vi "config CANcoder.vi"(8 "error in (no error)":errorcluster, 11 "CANcoder init data":T1={"description"="", "Installed?"=FALSE, "CAN ID"=0, "CAN Bus"="", "refnum name"="", "Sensor Direction"=FALSE, "Magnet Offset (Degrees)"=0.0, "gear ratio"=1.0} {"gear ratio" format="%_5f"}) -> (0 "error out":errorcluster)   [LabVIEW 2023]
uses:
  ctrl defs/ctrl CANcoder.ctl
  <vilib>/Rock Robotics/WPI/ThirdParty/Phoenix-LabVIEW/CANCoder/Controls/CTRE_Phoenix_CANcoder_Configurables.ctl
  <vilib>/Rock Robotics/WPI/ThirdParty/Phoenix-LabVIEW/CANCoder/Controls/CTRE_Phoenix_CANcoder_SensorInitializationStrategy.ctl
  <vilib>/Rock Robotics/WPI/ThirdParty/Phoenix-LabVIEW/CANCoder/Controls/CTRE_Phoenix_CANcoder_AbsoluteSensorRange.ctl
  <vilib>/Rock Robotics/WPI/ThirdParty/Phoenix-LabVIEW/Motor Controller/Controls/CTRE_Phoenix_MotorControl_VelocityMeasurementPeriod.ctl
  <vilib>/Rock Robotics/WPI/ThirdParty/Phoenix-LabVIEW/CANCoder/Controls/CTRE_Phoenix_CANcoder_SensorTimeBase.ctl
  <vilib>/Rock Robotics/WPI/ThirdParty/Phoenix-LabVIEW/CANCoder/Set/CTRE_Phoenix_CANcoder_SetPositionToAbsolute.vi
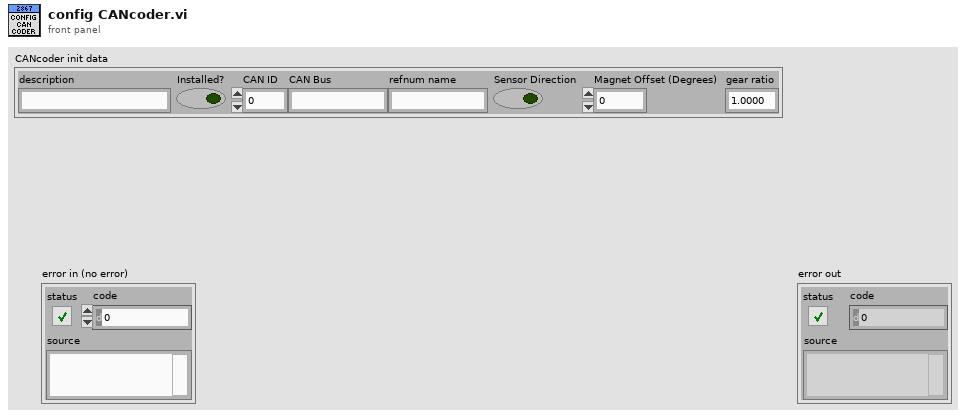
[diagram p1: front panel]
types:
  T1 = typedef "ctrl CANcoder.ctl" = cluster{"description":string, "Installed?":bool, "CAN ID":u8, "CAN Bus":string, "refnum name":string, "Sensor Direction":bool, "Magnet Offset (Degrees)":dbl, "gear ratio":dbl}
  T2 = typedef "CTRE_Phoenix_CANcoder_Configurables.ctl" = cluster{"Sensor Initialization Strategy":T3, "Absolute Sensor Range":T4, "Velocity Measurement Period":T5, "Velocity Measurement Window":i32, "Magnet Offset (Degrees)":dbl, "Sensor Direction":bool, "Sensor Coefficient":dbl, "Unit String":string, "Sensor Time Base":T6}
  T3 = typedef "CTRE_Phoenix_CANcoder_SensorInitializationStrategy.ctl" = enum16{"Boot To Zero", "Boot To Absolute Position"}
  T4 = typedef "CTRE_Phoenix_CANcoder_AbsoluteSensorRange.ctl" = enum16{"Unsigned [0 to 360)", "Signed [-180 to +180)"}
  T5 = typedef "CTRE_Phoenix_MotorControl_VelocityMeasurementPeriod.ctl" = u16
  T6 = typedef "CTRE_Phoenix_CANcoder_SensorTimeBase.ctl" = enum16{"Per100Ms_Legacy", "PerSecond", "PerMinute"}
  T7 = typedef "CTRE_Phoenix_CANcoder_DeviceRef.ctl" = cluster{"DeviceStatus":errorcluster, "Device Number":u8, "Handle":u64, "UsageFrame":u32, "Library Path":path}
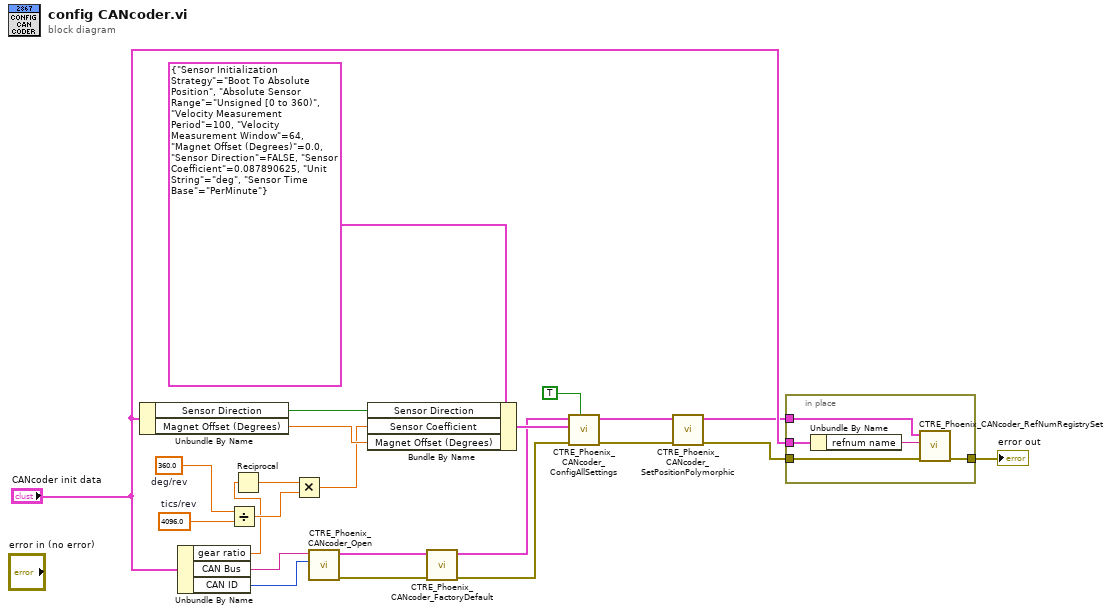
[diagram p0: block diagram]
diagram:
  w6 = 4096.0  # tics/rev
  w7 = 360.0  # deg/rev
  n1 = Unbundle By Name("CANcoder init data") -> ("Sensor Direction"=w16:bool, "Magnet Offset (Degrees)"=w15:dbl)
  n2 = Unbundle By Name("CANcoder init data") -> ("gear ratio"=w4:dbl, "CAN Bus"=w1:string, "CAN ID"=w2:u8)
  n3 = Divide(x=w7, y=w6) -> (x/y=w5:dbl)
  n4 = Reciprocal(x=w4) -> (1/x=w8:dbl)
  n5 = Multiply(x=w8, y=w5) -> (x*y=w3:dbl)
  n6 = call <vilib>:"CTRE_Phoenix_CANcoder_Open.vi"("Device Number"=w2, "CAN Bus"=w1) -> ("error out"=w22:errorcluster, "CTRE_CANcoder_DeviceRef"=w23:T7)  [unwired: 8 in]
  n7 = Bundle By Name(cluster=T2 {"Sensor Initialization Strategy"=enum."Boot To Absolute Position", "Absolute Sensor Range"=enum."Unsigned [0 to 360)", "Velocity Measurement Period"=100, "Velocity Measurement Window"=64, "Magnet Offset (Degrees)"=0.0, "Sensor Direction"=FALSE, "Sensor Coefficient"=0.087890625, "Unit String"="deg", "Sensor Time Base"=enum."PerMinute"} ("CANcoder Configurables"), "Sensor Direction"=w16, "Sensor Coefficient"=w3, "Magnet Offset (Degrees)"=w15) -> (w17:T2)
  n8 = call <vilib>:"CTRE_Phoenix_CANcoder_FactoryDefault.vi"("error in"=w22, "CTRE_CANcoder_DeviceRef"=w23) -> ("error out"=w13:errorcluster, "CTRE_CANcoder_DeviceRef"=w14:T7)  [unwired: 8 in]
  n9 = call <vilib>:"CTRE_Phoenix_CANcoder_ConfigAllSettings.vi"("Force Write"=TRUE, "error in (no error)"=w13, "CANcoder Configurables"=w17, "CTRE_CANcoder_DeviceRef"=w14) -> ("error out"=w11:errorcluster, "CTRE_CANcoder_DeviceRef"=w12:T7)  [unwired: 6 in]
  n10 = call-poly <vilib>:"CTRE_Phoenix_CANcoder_SetPositionPolymorphic.vi"("error in (no error)"=w11, "CTRE_CANcoder_DeviceRef"=w12) -> ("error out"=w9:errorcluster, "CTRE_CANcoder_DeviceRef"=w10:T7)  [unwired: 8 in]
  n11 = in-place {
    in-place-border: [w27] -> w21
    in-place-border: "CANcoder init data" -> [w26]
    in-place-border: w10 -> [w25]
    in-place-border: w9 -> [w24]
    n12 = Unbundle By Name(w26) -> ("refnum name"=w28:string)
    n13 = call <vilib>:"CTRE_Phoenix_CANcoder_RefNumRegistrySet.vi"("error in (no error)"=w24, "refnum name"=w28, "CTRE_CANcoder_DeviceRef"=w25) -> ("error out"=w27:errorcluster)  [unwired: 7 in, 1 out]
  }
  "error out" <- w21
